vi "ApplicationsSettings.vi"(8 "ErrorIn":errorcluster, 9 "Set default thresholds? [F]":bool) -> (0 "ErrorOut":errorcluster)   [LabVIEW 2019]
uses:
  MobileAnalyzer/mainVIs/aquireAccelerationDataVIs/Accelerometer.ctl
  FilePathToSaveAction.ctl
  MobileAnalyzer/mainVIs/analyzeAccelerationDataVIs/calculateFaultIndicatorsVIs/FaultParameter.ctl
  MobileAnalyzer/mainVIs/utilities/FGVAction.ctl
  MobileAnalyzer/mainVIs/analyzeAccelerationDataVIs/calculateFaultIndicatorsVIs/Thresholds.ctl
  AnalysisSettings.ctl
panel:
  in  "ParametersTab":enum32{"T", "F", "O"}(tab)
  in  "Kurtoza":dbl=5.0 min=0.0
  in  "RMS":dbl=0.3 min=0.0
  in  "Wsp. szczytu":dbl=0.3 min=0.0
  in  "Częstotliwości [Hz] i progi":dbl[][](array[numeric])=[[50.0, 0.5]] min=0.0
  in  "Szerokość filtrów pasmowych [%]":i32(slide)=20 scale=0.0..100.0
  in  "L. obrotów na znacznik":u16=1
  in  "Włączyć analizę rzędów?":bool
  in  "Nr rzędu i wartość progu":dbl[][](array[numeric])=[[1.0, 0.5], [4.0, 0.5], [7.0, 0.5]] min=0.0
  in  "ReadAnalysisSettings":bool
  in  "SaveAnalysisSettings":bool
  in  "Czestotliwość próbkowania [Hz]":dbl=4000.0 min=0.0
  in  "Wybierz akcelerometr:":T1=enum."MMA7351"
  in  "Zapisywać wyniki analizy?":bool
  in  "Zapisywać sygnały?":bool
  in  "Index":u32
  in  "DirPath":path
  in  "Seria pomiarowa":string="pomiar"
  in  "Close":bool
  # "Ustaw wartości progów parametrów:"
  # "Opis kategorii parametrów:\n   T - parametry w dziedzinie czasu\n   F - parametry w dziedzinie częstotliwości\n   O - analiza rzędów"
  # "Ustawienia analizatora:"
  # "Ustawienia aplikacji PC:"
  # "Wybierz ścieżkę do folderu na zapis sygnałów:"
  # "Podaj nr indeksu plików, od którego rozpocznie się numeracja.\nUwaga! Jeśli istnieje już plik z daną nazwą i podanym numerem \nindeksu, istniejący plik zostanie nadpisany."
  # "Nazwa serii pomiarowej - wspólna dla danych \nw analizatorze i aplikacji PC."
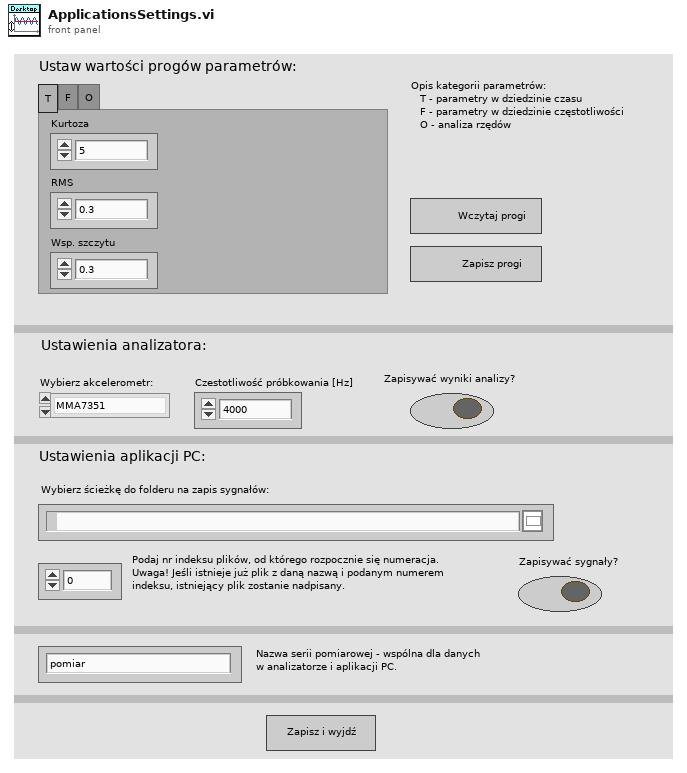
[diagram p1: front panel]
types:
  T1 = typedef "Accelerometer.ctl" = enum16{"None", "MPU6050", "MMA7351"}
  T2 = typedef "FilePathToSaveAction.ctl" = enum16{"Build new path", "Update index", "Get file path", "Get current settings"}
  T3 = typedef "FGVAction.ctl" = enum16{"Read", "Write"}
  T4 = enum16{"open", "replace", "create", "open or create", "replace or create", "replace or create with confirmation"}
  T5 = typedef "Thresholds.ctl" = cluster{"Parameters labels":T6[], "Parameters thresholds":dbl[], "Freqs and thresholds":dbl[][], "Orders and thresholds":dbl[][]}
  T6 = typedef "FaultParameter.ctl" = enum16{"Kurtosis", "RMS", "Crest factor"}
  T7 = typedef "AnalysisSettings.ctl" = cluster{"Fault Thresholds":T5, "Analysis series name":string, "Save data analysis?":bool, "Band size":i32, "OrderAnalysis?":bool, "Accelerometer":T1, "fs [Hz]":dbl, "Pulse per revolution":u16}
  T8 = typedef "DesktopAppSettings.ctl" = cluster{"MobileAnalyzer IP":string, "Network Stream Timeout Code":i32, "Endpoint Destroyed Code":i32, "Save to file?":bool, "All threads":T9[], "Connected":bool, "AnalysisSettings":T7}
  T9 = typedef "Thread.ctl" = enum16{"GUI", "communicateWithAnalyzer", "saveDataToTDMS"}
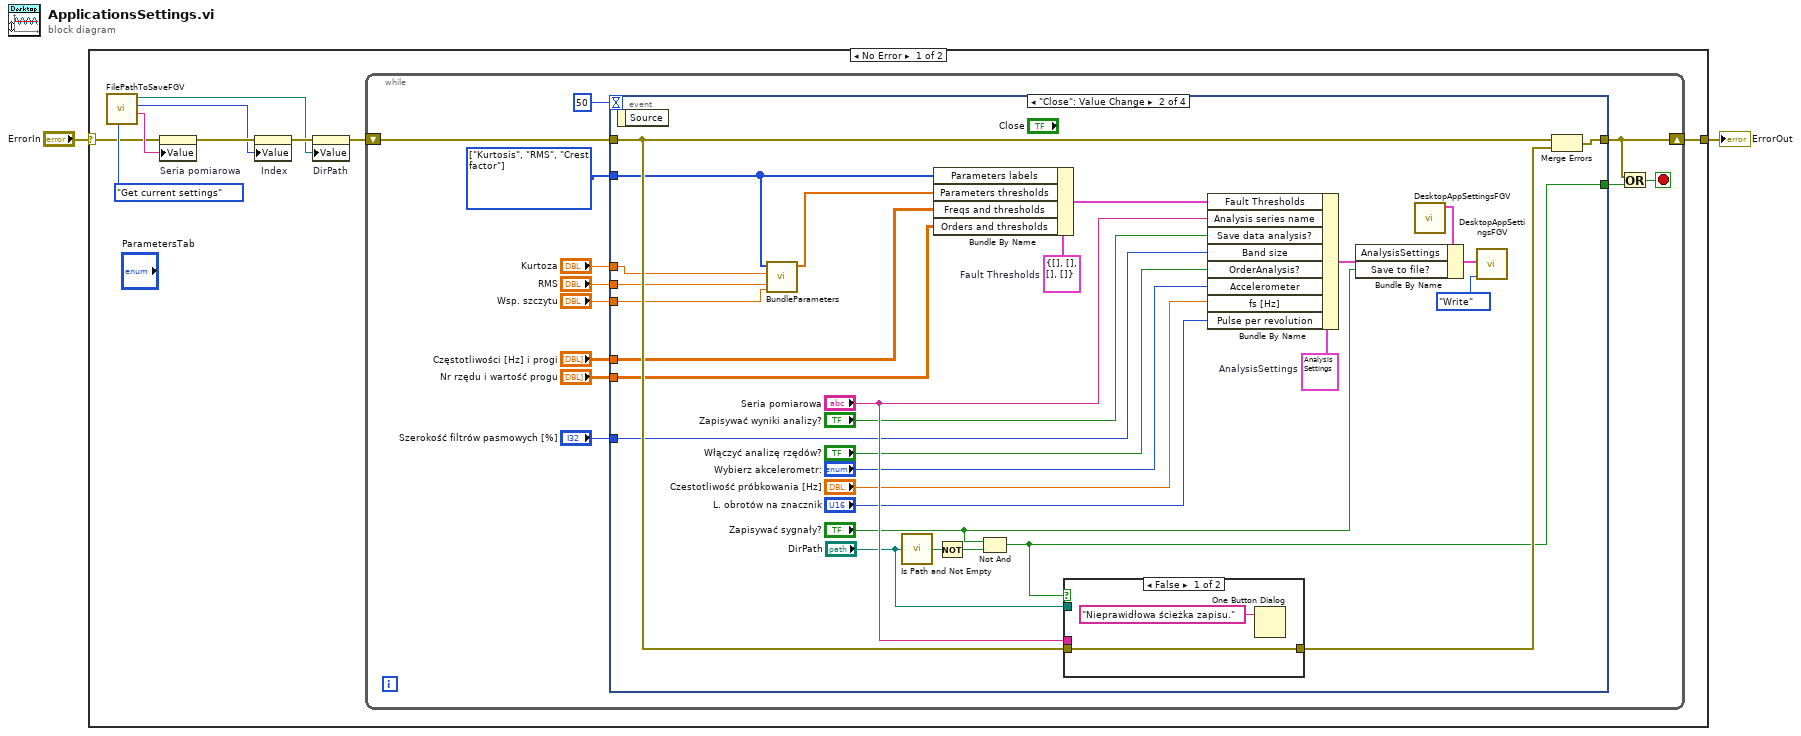
[diagram p0: block diagram]
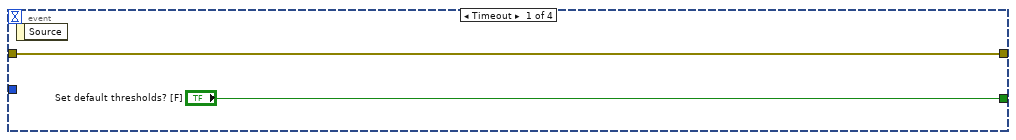
[diagram p2: hidden frame]
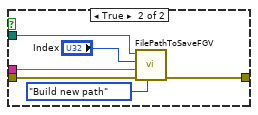
[diagram p3: hidden frame]
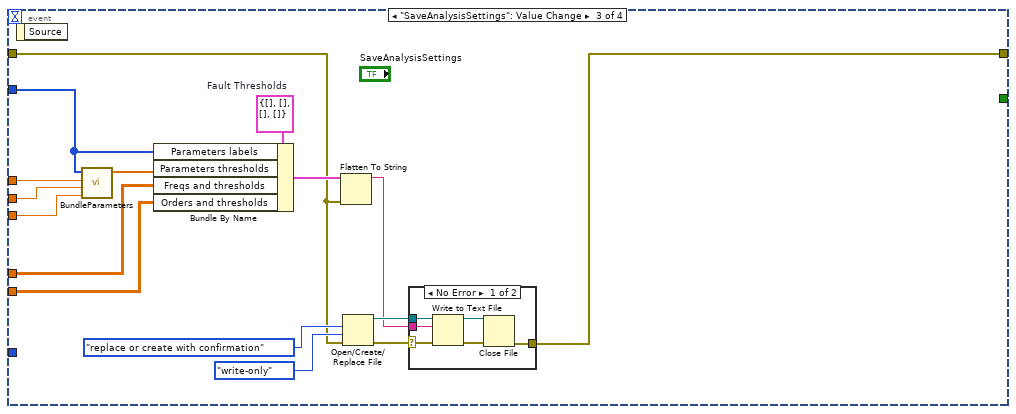
[diagram p4: hidden frame]
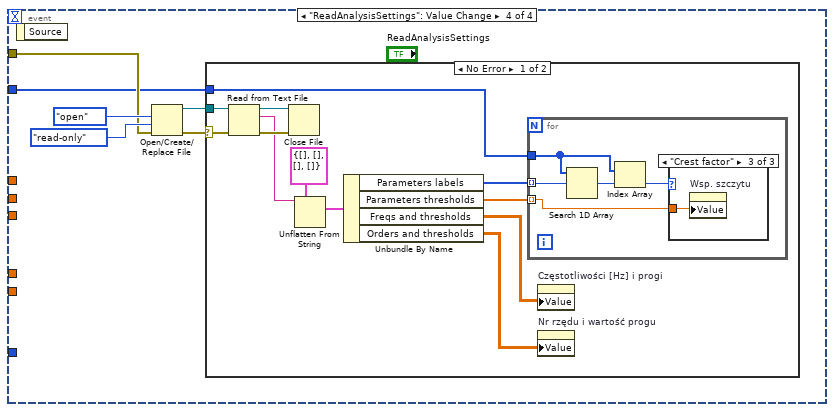
[diagram p6: hidden frame]
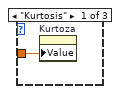
[diagram p7: hidden frame]
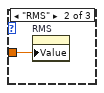
[diagram p8: hidden frame]
diagram:
  n1 = case shown="No Error" "ErrorIn" {
    selector: "ErrorIn" -> [w4 w112]
    tunnel: [w11 w112] -> w1
    frame No Error {
      n2 = call "FilePathToSaveFGV.vi"("FilePathToSaveAction"=FilePathToSaveAction."Get current settings") -> ("FileNamesOut"=w6:string, "IndexOut"=w8:u32, "File path"=w7:path)  [unwired: 7 in, 1 out]
      n3 = property on="Seria pomiarowa" class="Str"(error in=w4, "Value"=w6) -> (error out=w9:errorcluster)  [unwired: 1 in, 1 out]
      n4 = property on="Index" class="DigNum (strict)"(error in=w9, "Value"=w8) -> (error out=w10:errorcluster)  [unwired: 1 in, 1 out]
      n5 = property on="DirPath" class="Path"(error in=w10, "Value"=w7) -> (error out=w3:errorcluster)  [unwired: 1 in, 1 out]
      n6 = while {
        shift-right: [w19] -> w11
        shift-left: w3 -> [w20]
        stop <- w23 stop-if-true
        w12 = T6[] [enum."Kurtosis", enum."RMS", enum."Crest factor"] items=["Kurtosis", "RMS", "Crest factor"]
        n7 = event shown="[1] \"Close\": Value Change" {
          selector: _ -> [_ _ _ _]
          dyn-events: _ -> [_ _ _ _]
          timeout: 50 -> [_ _ _ _]
          tunnel: ["Set default thresholds? [F]" w26 _ _] -> w21
          tunnel: w20 -> [w24 w39 w64 w88]
          tunnel: [w24 w38 w65 _] -> w19
          tunnel: "Nr rzędu i wartość progu" -> [_ w37 w72 _]
          tunnel: "Częstotliwości [Hz] i progi" -> [_ w36 w71 _]
          tunnel: "Kurtoza" -> [_ w35 w77 _]
          tunnel: "RMS" -> [_ w34 w75 _]
          tunnel: "Wsp. szczytu" -> [_ w31 w76 _]
          tunnel: "Szerokość filtrów pasmowych [%]" -> [_ w33 _ _]
          tunnel: w12 -> [_ w32 w73 w86]
          event Timeout {
            n8 = event-data() -> ()  [unwired: 1 in, 1 out]
          }
          event "Close": Value Change {
            w42 = T7 {"Fault Thresholds"={"Parameters labels"=[], "Parameters thresholds"=[], "Freqs and thresholds"=[], "Orders and thresholds"=[]}, "Analysis series name"="Analiza", "Save data analysis?"=TRUE, "Band size"=20, "OrderAnalysis?"=FALSE, "Accelerometer"=enum."MPU6050", "fs [Hz]"=2000.0, "Pulse per revolution"=0}  # AnalysisSettings
            w40 = T5 {"Parameters labels"=[], "Parameters thresholds"=[], "Freqs and thresholds"=[], "Orders and thresholds"=[]}  # Fault Thresholds
            n9 = event-data() -> ()  [unwired: 1 in, 1 out]
            n10 = call "BundleParameters.vi"("Wsp. szczytu"=w31, "RMS"=w34, "Kurtoza"=w35, "Parameters labels"=w32) -> ("Parameters"=w45:dbl[])  [unwired: 7 in]
            n11 = call <vilib>:"Is Path and Not Empty.vi"("path"="DirPath") -> ("Is Path and Not Empty?"=w29:bool)  [unwired: 4 in]
            n12 = Bundle By Name(cluster=w40, "Parameters labels"=w32, "Parameters thresholds"=w45, "Freqs and thresholds"=w36, "Orders and thresholds"=w37) -> (w46:T5)
            n13 = Not(x=w29) -> (.not. x?=w28:bool)
            n14 = Not And(1:w28, 2:"Zapisywać sygnały?") -> (0:w26:bool)
            n15 = case shown="False" w26 {
              tunnel: w39 -> [w56 w62]
              tunnel: [w56 w61] -> w52
              tunnel: "DirPath" -> [_ w59]
              tunnel: "Seria pomiarowa" -> [_ w57]
              frame False {
                n16 = One Button Dialog(message="Nieprawidłowa ścieżka zapisu.") -> ()  [unwired: 1 in, 1 out]
              }
              frame True {
                n17 = call "FilePathToSaveFGV.vi"("FilePathToSaveAction"=FilePathToSaveAction."Build new path", "ErrorIn"=w62, "FilesNames"=w57, "Index"="Index", "DirPath"=w59) -> ("ErrorOut"=w61:errorcluster)  [unwired: 3 in, 3 out]
              }
            }
            n18 = Bundle By Name(cluster=w42, "Fault Thresholds"=w46, "Analysis series name"="Seria pomiarowa", "Save data analysis?"="Zapisywać wyniki analizy?", "Band size"=w33, "OrderAnalysis?"="Włączyć analizę rzędów?", "Accelerometer"="Wybierz akcelerometr:", "fs [Hz]"="Czestotliwość próbkowania [Hz]", "Pulse per revolution"="L. obrotów na znacznik") -> (w47:T7)
            n19 = call "DesktopAppSettingsFGV.vi"() -> ("DesktopAppSettingsOut"=w43:T8)  [unwired: 11 in]
            n20 = Bundle By Name(cluster=w43, "AnalysisSettings"=w47, "Save to file?"="Zapisywać sygnały?") -> (w44:T8)
            n21 = call "DesktopAppSettingsFGV.vi"("FGVAction (Read)"=FGVAction."Write", "DesktopAppSettingsIn"=w44) -> ()  [unwired: 9 in, 1 out]
            n22 = Merge Errors(w39, w52) -> (w38:errorcluster)
          }
          event "SaveAnalysisSettings": Value Change {
            w78 = T5 {"Parameters labels"=[], "Parameters thresholds"=[], "Freqs and thresholds"=[], "Orders and thresholds"=[]}  # Fault Thresholds
            n23 = event-data() -> ()  [unwired: 1 in, 1 out]
            n24 = call "BundleParameters.vi"("Wsp. szczytu"=w76, "RMS"=w75, "Kurtoza"=w77, "Parameters labels"=w73) -> ("Parameters"=w74:dbl[])  [unwired: 7 in]
            n25 = Bundle By Name(cluster=w78, "Parameters labels"=w73, "Parameters thresholds"=w74, "Freqs and thresholds"=w71, "Orders and thresholds"=w72) -> (w70:T5)
            n26 = Flatten To String(anything=w70, error in (no error)=w64) -> (data string=w66:string)  [unwired: 2 in, 2 out]
            n27 = Open/Create/Replace File(error in=w64, operation (0:open)=T4."replace or create with confirmation", access (0:read/write)=enum16{"read/write", "read-only", "write-only"}."write-only") -> (refnum out=w67:refnum<file>, error out=w63:errorcluster)  [unwired: 3 in, 1 out]
            n28 = case shown="No Error" w63 {
              selector: w63 -> [w79 w85]
              tunnel: w67 -> [w84 _]
              tunnel: w66 -> [w83 _]
              tunnel: [w80 w85] -> w65
              frame No Error {
                n29 = Write to Text File(file (use dialog)=w84, text=w83, error in=w79) -> (refnum out=w82:refnum<file>, error out=w81:errorcluster)  [unwired: 1 in, 1 out]
                n30 = Close File(refnum=w82, error in=w81) -> (error out=w80:errorcluster)  [unwired: 1 out]
              }
              frame Error {
              }
            }
          }
          event "ReadAnalysisSettings": Value Change {
            n31 = event-data() -> ()  [unwired: 1 in, 1 out]
            n32 = Open/Create/Replace File(error in=w88, operation (0:open)=T4."open", access (0:read/write)=enum16{"read/write", "read-only", "write-only"}."read-only") -> (refnum out=w91:refnum<file>, error out=w87:errorcluster)  [unwired: 3 in, 1 out]
            n33 = case shown="No Error" w87 {
              selector: w87 -> [w103 _]
              tunnel: w91 -> [w102 _]
              tunnel: w86 -> [w95 _]
              frame No Error {
                n34 = Read from Text File(file (use dialog)=w102, error in=w103) -> (refnum out=w101:refnum<file>, text=w98:string, error out=w100:errorcluster)  [unwired: 2 in, 1 out]
                n35 = Close File(refnum=w101, error in=w100) -> ()  [unwired: 2 out]
                n36 = Unflatten From String(type=T5 {"Parameters labels"=[], "Parameters thresholds"=[], "Freqs and thresholds"=[], "Orders and thresholds"=[]} ("Fault Thresholds"), binary string=w98) -> (value=w97:T5)  [unwired: 3 in, 2 out]
                n37 = Unbundle By Name(w97) -> ("Parameters labels"=w96:T6[], "Parameters thresholds"=w94:dbl[], "Freqs and thresholds"=w93:dbl[][], "Orders and thresholds"=w92:dbl[][])
                n38 = for {
                  tunnel: w96 -> [w108] mode=indexing
                  tunnel: w95 -> [w107]
                  tunnel: w94 -> [w104] mode=indexing
                  n39 = Search 1D Array(1D array=w107, element=w108) -> (index of element=w106:i32)  [unwired: 1 in]
                  n40 = Index Array(array=w107, index=w106) -> (element=w105:T6)
                  n41 = case shown="\"Crest factor\"" w105 {
                    tunnel: w104 -> [w109 w110 w111]
                    frame "Kurtosis" {
                      n42 = property on="Kurtoza" class="DigNum (strict)"("Value"=w109) -> ()  [unwired: 2 in, 2 out]
                    }
                    frame "RMS" {
                      n43 = property on="RMS" class="DigNum (strict)"("Value"=w110) -> ()  [unwired: 2 in, 2 out]
                    }
                    frame "Crest factor" {
                      n44 = property on="Wsp. szczytu" class="DigNum (strict)"("Value"=w111) -> ()  [unwired: 2 in, 2 out]
                    }
                  }
                }
                n45 = property on="Częstotliwości [Hz] i progi" class="Arr (strict)"("Value"=w93) -> ()  [unwired: 2 in, 2 out]
                n46 = property on="Nr rzędu i wartość progu" class="Arr (strict)"("Value"=w92) -> ()  [unwired: 2 in, 2 out]
              }
              frame Error {
              }
            }
          }
        }
        n47 = Or(x=w19, y=w21) -> (x .or. y?=w23:bool)
      }
    }
    frame Error {
    }
  }
  "ErrorOut" <- w1
